vi "DAC Stop.vi"(8 "error in (no error)":errorcluster, 11 "DAC Traverse in":refnum<class "DAC Traverse.lvclass">) -> (0 "error out":errorcluster, 3 "DAC Traverse out":refnum<class "DAC Traverse.lvclass">)   [LabVIEW 2019, in "DAC.lvlib" / "DAC Traverse.lvclass"]
uses:
  DAC Traverse.lvclass
  C:/Users/wg/Documents/LV_Projects/test-stand/App/DAC/DAC.lvclass
  DAC.lvclass/DAC.ctl
  DAC Traverse.lvclass/DAC Traverse.ctl
  DAC.lvclass
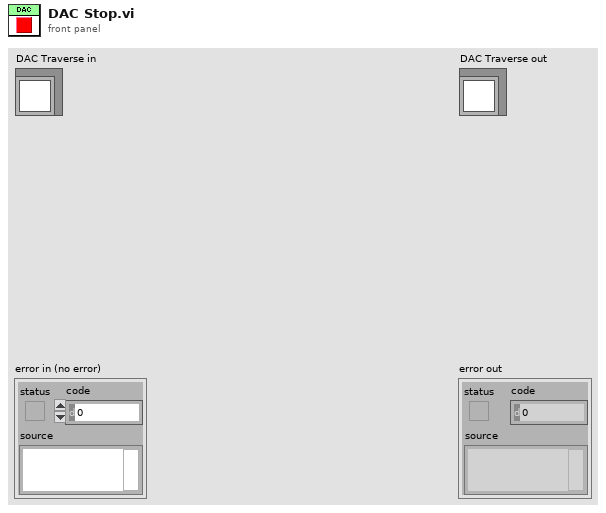
[diagram p1: front panel]
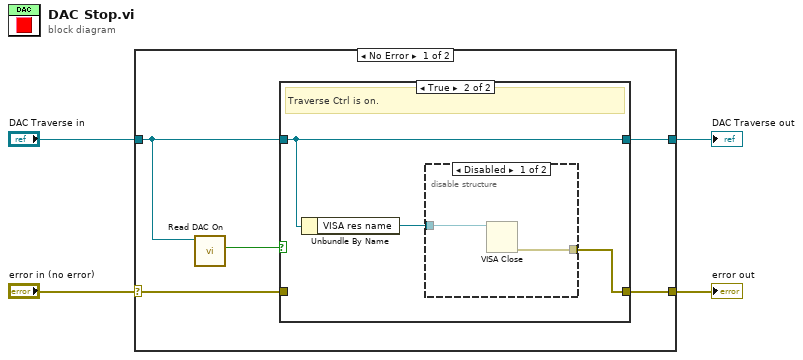
[diagram p0: block diagram]
diagram:
  n1 = case shown="No Error" "error in (no error)" {
    selector: "error in (no error)" -> [w6 w18]
    tunnel: [w5 w18] -> w1
    tunnel: [w7 w17] -> w3
    tunnel: "DAC Traverse in" -> [w9 w17]
    frame No Error {
      n2 = call "Read DAC On.vi"("DAC in"=w9) -> ("DAC On"=w8:bool)  [unwired: 8 in, 2 out]
      n3 = case shown="True" w8 {
        tunnel: w9 -> [w11 w14]
        tunnel: [w11 w14] -> w7
        tunnel: w6 -> [w10 _]
        tunnel: [w10 w12] -> w5
        frame False {
          # "Traverse Ctrl is off."
        }
        frame True {
          # "Traverse Ctrl is on."
          n4 = Unbundle By Name(w14) -> ("VISA res name"=w13:refnum<visa-resource-name>)
          n5 = disable-structure shown="Disabled" {
            disable-tunnel: w13 -> [w16 _]
            disable-tunnel: [w15 _] -> w12
            frame Disabled {
              n6 = VISA Close(VISA resource name=w16) -> (error out=w15:errorcluster)  [unwired: 1 in]
            }
            frame Enabled {
            }
          }
        }
      }
    }
    frame Error {
    }
  }
  "error out" <- w1
  "DAC Traverse out" <- w3
